vi "PQueue Pop.vi"(11 "PQueue in":T1[](array[typedef])) -> (2 "Path":T1, 3 "PQueue out":T1[](array[typedef]))   [LabVIEW 2017]
uses:
  Path.ctl
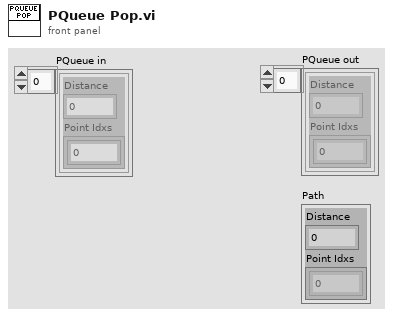
[diagram p1: front panel]
types:
  T1 = typedef "Path.ctl" = cluster{"Distance":dbl, "Point Idxs":i32[]}
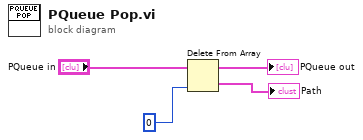
[diagram p0: block diagram]
diagram:
  n1 = Delete From Array(array="PQueue in", index=0) -> (deleted portion=→"Path":T1, array with subset deleted=→"PQueue out":T1[])  [unwired: 1 in]
